vi "17mart 2.vi"() -> ()   [LabVIEW 2020]
panel:
  in  "Numeric":i32
  out "p-2":dbl
  out "p-1":dbl
  out "p":dbl
  out "p-1":dbl
  out "i":i32
  out "slay 2":dbl
  out "cont 2":dbl
  out "Boolean 2":bool
  in  "deneme tf":bool
  in  "deneme":dbl
  out "output cluster 2":cluster{"bla":dbl, "Boolean":bool}
  out "output cluster":cluster{"Numeric":dbl, "Boolean":bool}
  in  "Boolean":bool
  in  "slay":dbl
  in  "Cluster":T1
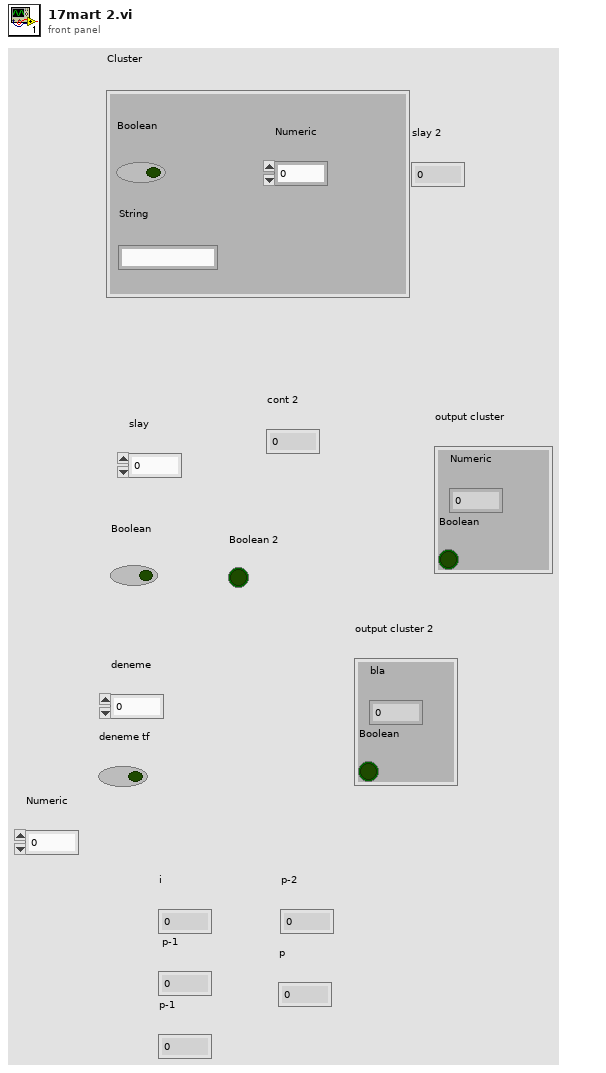
[diagram p1: front panel]
types:
  T1 = cluster{"Numeric":dbl, "Boolean":bool, "String":string}
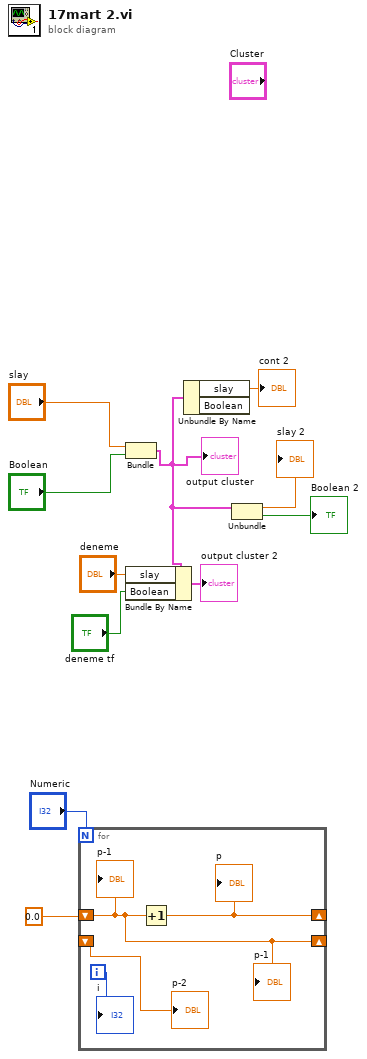
[diagram p0: block diagram]
diagram:
  n1 = for {
    N: "Numeric" -> [_]
    shift-right: [w15] -> _
    shift-left: 0.0 -> [w14]
    shift-right: [w14] -> _
    shift-left: _ -> [w12]
    i -> [w13]
    n2 = Increment(x=w14) -> (x+1=w15:dbl)
    "p" <- w15
    "i" <- w13
    "p-1" <- w14
    "p-1" <- w14
    "p-2" <- w12
  }
  n3 = Bundle("slay"="slay", "Boolean"="Boolean") -> (w5:cluster{"slay":dbl, "Boolean":bool})  [unwired: 1 in]
  "output cluster" <- w5
  n4 = Bundle By Name(cluster=w5, "slay"="deneme", "Boolean"="deneme tf") -> (→"output cluster 2":cluster{"slay":dbl, "Boolean":bool})
  n5 = Unbundle By Name(w5) -> ("slay"=→"cont 2":dbl)  [unwired: 1 out]
  n6 = Unbundle(w5) -> ("slay"=→"slay 2":dbl, "Boolean"=→"Boolean 2":bool)
